vi "Write Setpoint.vi"(8 "error in (no error)":errorcluster, 9 "Value":dbl, 10 "Variable":string, 11 "IED in":refnum<class "IED.lvclass">) -> (0 "error out":errorcluster, 3 "IED out":refnum<class "IED.lvclass">)   [LabVIEW 2015, in "IED Actor.lvlib" / "IED.lvclass"]
uses:
  IED.lvclass
  <vilib>/ActorFramework/Actor/Actor.lvclass/Actor.ctl
  IED.lvclass/IED.ctl
  SCADA Core/SCADA Abstract Messages/IED Setpoint Status Msg/IED Setpoint Status.ctl
  SCADA Core/SCADA Response Messages/Return Setpoint Status Msg/Return Setpoint Status Msg.lvclass/Return Setpoint Status Msg.ctl
  <vilib>/ActorFramework/Message Enqueuer/Message Enqueuer.lvclass/Message Enqueuer.ctl
  <vilib>/NI/Tools/Keyed Array/Map String.vi
  <vilib>/ActorFramework/Message Enqueuer/Enqueue.vi
  <vilib>/NI/Tools/String/Get Case Matching.vi
  <vilib>/ActorFramework/Message Priority Queue/Priority Enqueue.vi
  SCADA Core/SCADA Response Messages/Return Setpoint Status Msg/Return Setpoint Status Msg.lvclass
  <vilib>/Modbus/master/Modbus Master.lvclass
  <vilib>/NI/Tools/Keyed Array/Tools_KeyedArray.lvlib
  SCADA Core/SCADA Abstract Messages/IED Setpoint Status Msg/IED Setpoint Status Msg.lvclass
  <vilib>/ActorFramework/Actor/Actor.lvclass
  Utilities/Message Strings.llb/Message String Utilities.lvlib
  Utilities/Modbus Data Conversion.llb/Modbus Data Conversion.lvlib
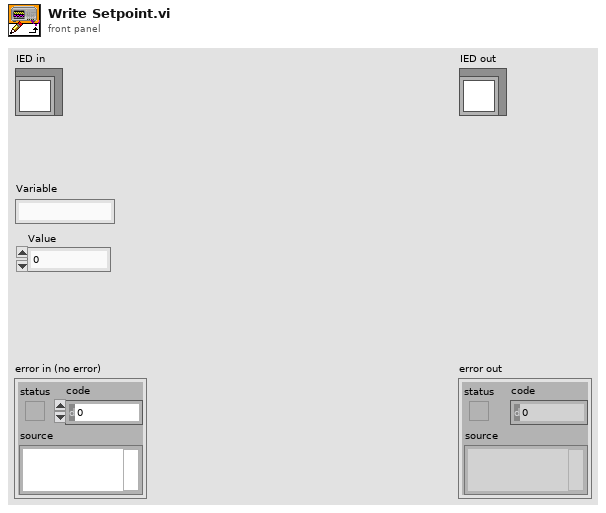
[diagram p1: front panel]
types:
  T1 = typedef "SCADA Core.lvlib/IED Setpoint Status Msg.lvclass/IED Setpoint Status.ctl" = enum16{"Success", "Failure", "Multiple Success", "Multiple Failure"}
  T2 = typedef "Tools_KeyedArray.lvlib/KeyedArray.ctl" = cluster{"keys":string[], "values":string[]}
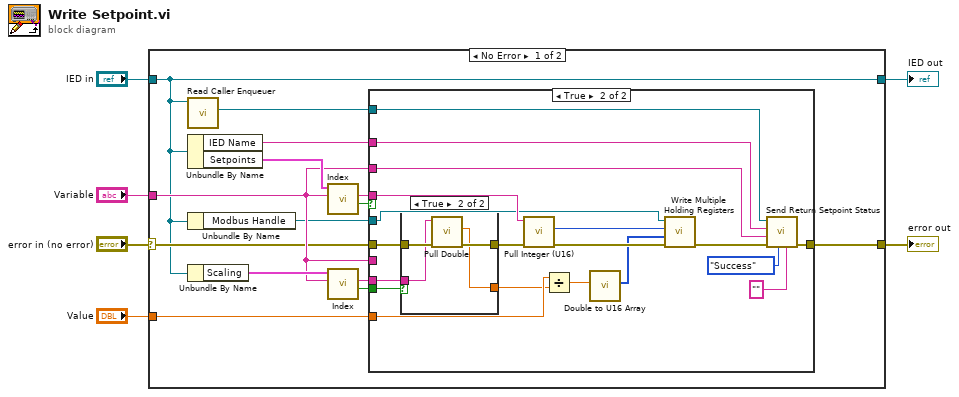
[diagram p0: block diagram]
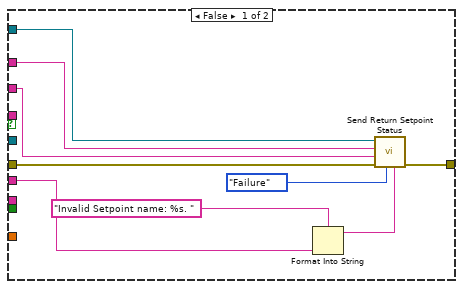
[diagram p2: hidden frame]
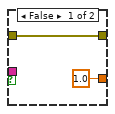
[diagram p3: hidden frame]
diagram:
  n1 = case shown="No Error" "error in (no error)" {
    selector: "error in (no error)" -> [w9 w56]
    tunnel: [w10 w56] -> w5
    tunnel: [w8 w55] -> w3
    tunnel: "IED in" -> [w8 w55]
    tunnel: "Variable" -> [w11 _]
    tunnel: "Value" -> [w18 _]
    frame No Error {
      n2 = call <vilib>:"Read Caller Enqueuer.vi"("Actor"=w8) -> ("Caller Enqueuer"=w16:refnum<class "Message Enqueuer.lvclass">)  [unwired: 10 in]
      n3 = Unbundle By Name(w8) -> ("IED Name"=w12:string, "Setpoints"=w20:T2)
      n4 = Unbundle By Name(w8) -> ("Modbus Handle"=w7:refnum<class "Modbus Master.lvclass">)
      n5 = Unbundle By Name(w8) -> ("Scaling"=w15:T2)
      n6 = call <vilib>:"Index.vi"("key"=w11, "array in"=w20) -> ("valid key"=w17:bool, "value"=w19:string)  [unwired: 3 in, 1 out]
      n7 = call <vilib>:"Index.vi"("key"=w11, "array in"=w15) -> ("valid key"=w14:bool, "value"=w13:string)  [unwired: 3 in, 1 out]
      n8 = case shown="True" w17 {
        tunnel: w19 -> [_ w42]
        tunnel: w18 -> [_ w37]
        tunnel: w9 -> [w28 w40]
        tunnel: [w29 w48] -> w10
        tunnel: w11 -> [w23 w47]
        tunnel: w16 -> [w27 w35]
        tunnel: w12 -> [w24 w36]
        tunnel: w14 -> [_ w31]
        tunnel: w13 -> [_ w38]
        tunnel: w11 -> [w21 _]
        tunnel: w7 -> [_ w34]
        frame False {
          n9 = Format Into String(format string="Invalid Setpoint name: %s. " ("Error String"), w21) -> (resulting string=w22:string)  [unwired: 2 in, 1 out]
          n10 = call "Send Return Setpoint Status.vi"("error"=w22, "Status"=IED_Setpoint_Status."Failure", "error in (no error)"=w28, "Setpoint Name"=w23, "IED Name"=w24, "Message Enqueuer"=w27) -> ("error out"=w29:errorcluster)  [unwired: 4 in, 1 out]
        }
        frame True {
          n11 = case shown="True" w31 {
            tunnel: w40 -> [w50 w54]
            tunnel: [w50 w53] -> w39
            tunnel: w38 -> [_ w52]
            tunnel: [1.0 ("Double out") w51] -> w30
            frame False {
            }
            frame True {
              n12 = call "Pull Double.vi"("error in (no error)"=w54, "String in"=w52) -> ("error out"=w53:errorcluster, "Double out"=w51:dbl)  [unwired: 7 in, 1 out]
            }
          }
          n13 = call "Pull Integer (U16).vi"("error in (no error)"=w39, "String in"=w42) -> ("error out"=w43:errorcluster, "Integer out"=w41:u16)  [unwired: 7 in, 1 out]
          n14 = Divide(x=w37, y=w30) -> (x/y=w33:dbl)
          n15 = call "Double to U16 Array.vi"("Double"=w33) -> ("U16 Array"=w32:u16[])  [unwired: 10 in]
          n16 = call-dynamic "Write Multiple Holding Registers.vi"("error in (no error)"=w43, "holding register values"=w32, "starting address"=w41, "Modbus master in"=w34) -> ("error out"=w44:errorcluster)  [unwired: 6 in, 1 out]
          n17 = call "Send Return Setpoint Status.vi"("error"="" ("Error String"), "Status"=IED_Setpoint_Status."Success", "error in (no error)"=w44, "Setpoint Name"=w47, "IED Name"=w36, "Message Enqueuer"=w35) -> ("error out"=w48:errorcluster)  [unwired: 4 in, 1 out]
        }
      }
    }
    frame Error {
    }
  }
  "error out" <- w5
  "IED out" <- w3
